vi "Read UI Refnum.vi"(8 "error in (no error)":errorcluster, 11 "ConfigureableObject in":refnum<class "CallVIStep.lvclass">) -> (0 "error out":errorcluster, 2 "VI Refnum":refnum<vi>, 3 "ConfigureableObject out":refnum<class "CallVIStep.lvclass">)   [LabVIEW 2015, in "CallVIStep.lvclass"]
uses:
  CallVIStep.lvclass
  VIStep Configure UI.vi
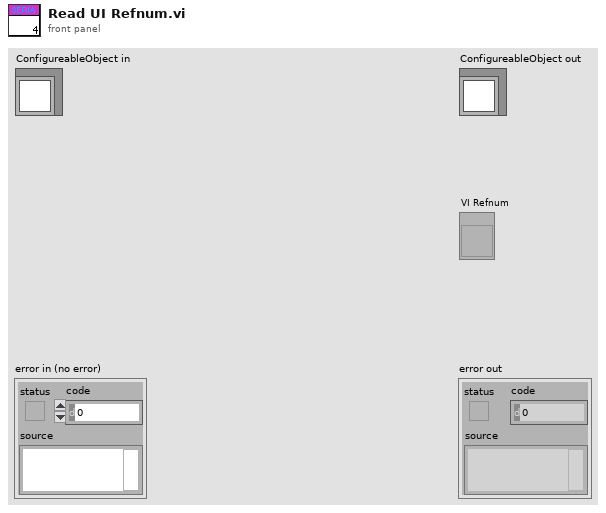
[diagram p1: front panel]
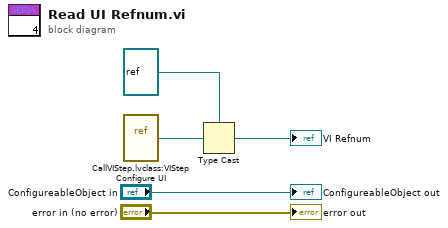
[diagram p0: block diagram]
diagram:
  n1 = vi-ref "CallVIStep.lvclass:VIStep Configure UI.vi"() -> (w3:refnum<vi>)
  n2 = Type Cast(type=refnum<vi> refnum ("vi reference"), x=w3) -> (*(type *) &x=→"VI Refnum":refnum<vi>)
  "error out" <- "error in (no error)"
  "ConfigureableObject out" <- "ConfigureableObject in"
